vi "Add items (bytes).vi"(10 "Array":u8[](array[numeric]), 11 "MsgPackArray in":refnum<class "MsgPackArray.lvclass">) -> (3 "MsgPackArray out":refnum<class "MsgPackArray.lvclass">)   [LabVIEW 2020, in "MessagePack.lvlib" / "MsgPackArray.lvclass"]
uses:
  MsgPackArray.lvclass
  Element.ctl
  MsgPackArray.lvclass/MsgPackArray.ctl
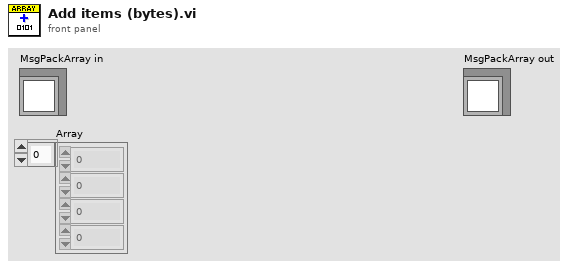
[diagram p1: front panel]
types:
  T1 = typedef "MessagePack.lvlib/MsgPackArray.lvclass/Element.ctl" = cluster{"element bytes":u8[]}
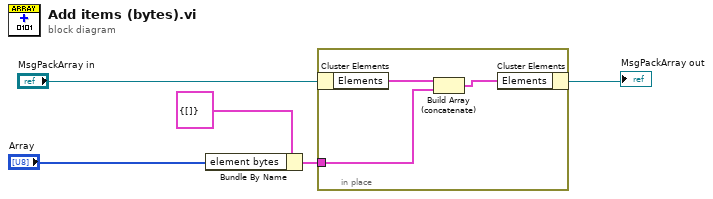
[diagram p0: block diagram]
diagram:
  n1 = Bundle By Name(cluster=T1 {"element bytes"=[]} ("Element"), "element bytes"="Array") -> (w1:T1)
  n2 = in-place {
    in-place-border: w1 -> [w7]
    n3 = in-place-cluster #1("MsgPackArray in") -> ("Elements"=w8:T1[])
    n4 = Build Array (concatenate)(w8, w7) -> (w6:T1[])
    n5 = in-place-cluster #1("Elements"=w6) -> (→"MsgPackArray out":refnum<class "MsgPackArray.lvclass">)
  }
